vi "Enqueue Message.vi"(8 "error in (no error)":errorcluster, 10 "output cluster":T1) -> (0 "error out":errorcluster, 3 "queue out":refnum<queue>)   [LabVIEW 2014, in "Control Module.lvlib"]
uses:
  Control Module.lvlib
  Message.ctl
  Queue FGV.ctl
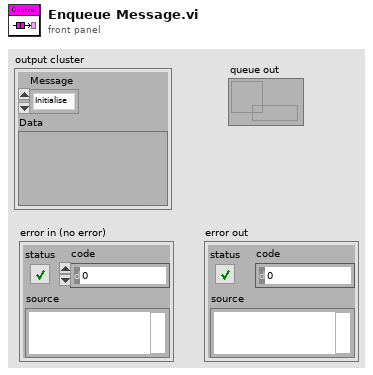
[diagram p1: front panel]
types:
  T1 = typedef "Control Module.lvlib/Message.ctl" = cluster{"Message":enum16{"Initialise", "Error", "Close"}, "Data":variant}
  T2 = typedef "Control Module.lvlib/Queue FGV.ctl" = enum16{"Set", "Get", "Release"}
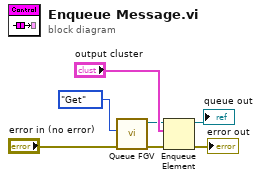
[diagram p0: block diagram]
diagram:
  n1 = call "Queue FGV.vi"("error in (no error)"="error in (no error)", "Action"=Queue_FGV."Get") -> ("error out"=w6:errorcluster, "Queue Out"=w2:refnum<queue>)  [unwired: 8 in]
  n2 = Enqueue Element(queue=w2, element="output cluster", error in (no error)=w6) -> (queue out=→"queue out":refnum<queue>, error out=→"error out":errorcluster)  [unwired: 1 in, 1 out]
